vi "Strings to Helium Configuration.vi"(10 "Thresholds":string[][](array[string]), 11 "Timings":string[][](array[string])) -> (2 "Thresholds":T1[](array[typedef]), 3 "Timings":T2[](array[typedef]))   [LabVIEW 2015]
uses:
  Tests/Controls/Test Timing.ctl
  Tests/Controls/Helium Thresholds.ctl
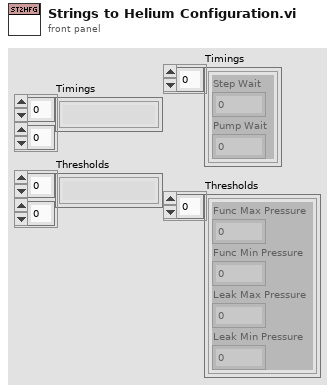
[diagram p1: front panel]
types:
  T1 = typedef "Helium Thresholds.ctl" = cluster{"Func Max Pressure":dbl, "Func Min Pressure":dbl, "Leak Max Pressure":dbl, "Leak Min Pressure":dbl}
  T2 = typedef "Test Timing.ctl" = cluster{"Step Wait":dbl, "Pump Wait":dbl}
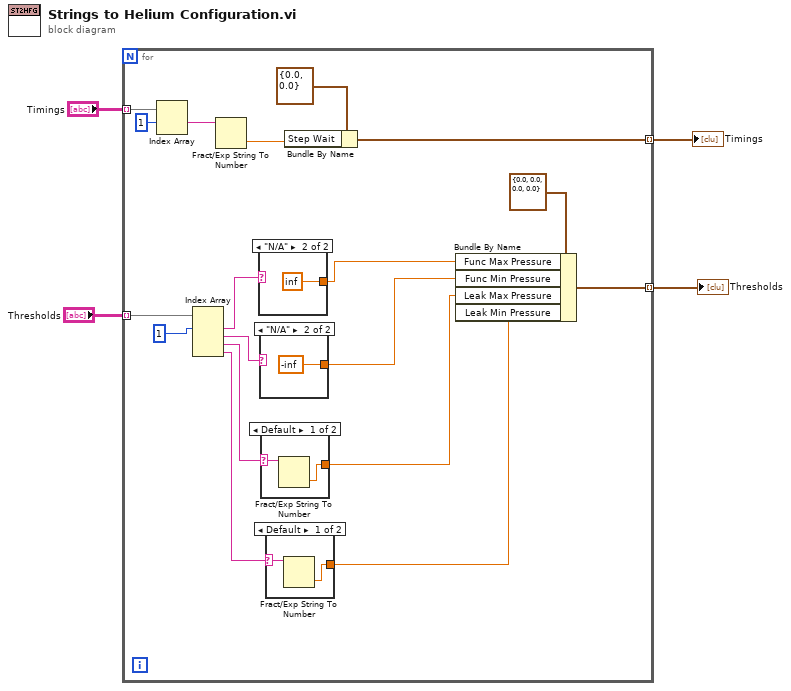
[diagram p0: block diagram]
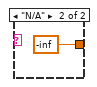
[diagram p2: hidden frame]
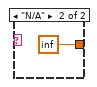
[diagram p3: hidden frame]
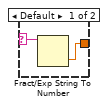
[diagram p4: hidden frame]
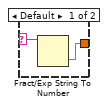
[diagram p5: hidden frame]
diagram:
  n1 = for {
    tunnel: "Timings" -> [w22] mode=indexing
    tunnel: "Thresholds" -> [w10] mode=indexing
    tunnel: [w18] -> w2 mode=indexing
    tunnel: [w17] -> w1 mode=indexing
    n2 = Index Array(array=w22, index #1=1 ("index")) -> (element #1=w20:string)  [unwired: 1 in, 1 out]
    n3 = Index Array(array=w10, index #1=1 ("index")) -> (element #1=w11:string, element #2=w12:string, element #3=w13:string, element #4=w14:string)  [unwired: 3 in]
    n4 = Fract/Exp String To Number(string=w20) -> (number=w19:dbl)  [unwired: 3 in, 1 out]
    n5 = case shown="\"N/A\"" w11 {
      selector: w11 -> [w33 _]
      tunnel: [w32 inf ("Func Max Pressure")] -> w9
      frame Default {
        n6 = Fract/Exp String To Number(string=w33) -> (number=w32:dbl)  [unwired: 3 in, 1 out]
      }
      frame "N/A" {
      }
    }
    n7 = case shown="\"N/A\"" w12 {
      selector: w12 -> [w30 _]
      tunnel: [w29 -inf ("Func Max Pressure")] -> w8
      frame Default {
        n8 = Fract/Exp String To Number(string=w30) -> (number=w29:dbl)  [unwired: 3 in, 1 out]
      }
      frame "N/A" {
      }
    }
    n9 = case shown="Default" w13 {
      selector: w13 -> [w27 _]
      tunnel: [w26 inf ("Func Max Pressure")] -> w7
      frame Default {
        n10 = Fract/Exp String To Number(string=w27) -> (number=w26:dbl)  [unwired: 3 in, 1 out]
      }
      frame "N/A" {
      }
    }
    n11 = case shown="Default" w14 {
      selector: w14 -> [w24 _]
      tunnel: [w23 -inf ("Func Max Pressure")] -> w6
      frame Default {
        n12 = Fract/Exp String To Number(string=w24) -> (number=w23:dbl)  [unwired: 3 in, 1 out]
      }
      frame "N/A" {
      }
    }
    n13 = Bundle By Name(cluster=T2 {"Step Wait"=0.0, "Pump Wait"=0.0} ("Timing"), "Step Wait"=w19) -> (w18:T2)
    n14 = Bundle By Name(cluster=T1 {"Func Max Pressure"=0.0, "Func Min Pressure"=0.0, "Leak Max Pressure"=0.0, "Leak Min Pressure"=0.0} ("Helium Thresholds"), "Func Max Pressure"=w9, "Func Min Pressure"=w8, "Leak Max Pressure"=w7, "Leak Min Pressure"=w6) -> (w17:T1)
  }
  "Timings" <- w2
  "Thresholds" <- w1
